vi "Initialize with Options.vi"(7 "Option string (\"\")":string, 8 "error in (no error)":errorcluster, 9 "Reset (T: Reset)":bool=TRUE, 10 "ID Query (T: Check)":bool=TRUE, 11 "VISA resource name":refnum<visa-resource-name>="TCPIP::192.168.5.120::INST") -> (0 "error out":errorcluster, 3 "VISA resource name out":refnum<visa-resource-name>)   [LabVIEW 2015, in "Rohde&Schwarz CMP LR WPAN Measurement.lvlib"]
doc: "This VI opens a new session to the instrument.\nCompared to the <b>Initialize.vi</b>, this one allows for additional settings in the <b>Option string</b>."
uses:
  <instrlib>/Rohde&Schwarz CMP LR WPAN Measurement/Rohde&Schwarz CMP LR WPAN Measurement.lvlib
  <instrlib>/Rohde&Schwarz CMP LR WPAN Measurement/Private/rsidr_core.llb/type_Session_Parameter_int32.ctl
  <instrlib>/Rohde&Schwarz CMP LR WPAN Measurement/Private/rsidr_core.llb/type_Session_Parameter_Boolean.ctl
  <instrlib>/Rohde&Schwarz CMP LR WPAN Measurement/Public/Utility/rsidr_core_global.vi
  <instrlib>/Rohde&Schwarz CMP LR WPAN Measurement/Private/rsidr_core.llb/rsidr_core.lvlib
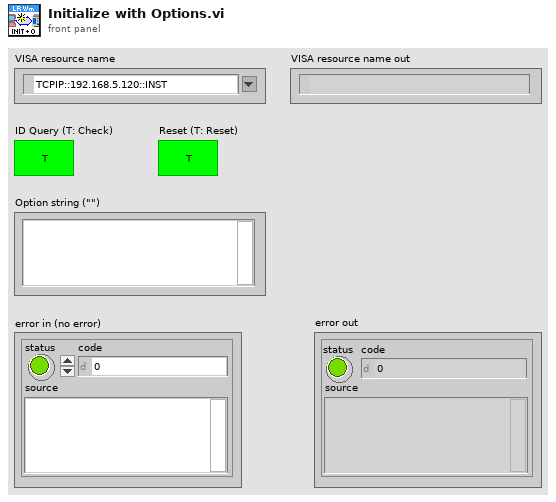
[diagram p1: front panel]
types:
  T1 = typedef "Rohde&Schwarz CMP LR WPAN Measurement.lvlib/rsidr_core.lvlib/type_Session_Parameter_Boolean.ctl" = enum16{"Simulate", "Query Instr Status", "Check Range", "Check Options", "Add LF to Write", "Duplicate Session", "Fast Sweep", "Logging", "OPC-sync Attribute Queries", "OPC-sync Attribute Writes"}
  T2 = typedef "Rohde&Schwarz CMP LR WPAN Measurement.lvlib/rsidr_core.lvlib/type_Session_Parameter_int32.ctl" = enum16{"OPC Timeout", "Additional Flags", "Wait Before Write", "Wait Before Read", "Bin Data Chunk Size", "VISA Access Mode", "VISA Timeout", "Bin Float Number Format", "Bin Integer Number Format", "STBpollVISAtimeout", "OPCwaitMode"}
  T3 = typedef "Rohde&Schwarz CMP LR WPAN Measurement.lvlib/rsidr_core.lvlib/type_Input_Format_RepCap.ctl" = cluster{"repCapName":string, "indetifiers":string[], "cmdValues":string[]}
  T4 = typedef "Rohde&Schwarz CMP LR WPAN Measurement.lvlib/rsidr_core.lvlib/type_Input_Format_RangeTable.ctl" = cluster{"Type":u16, "Name":string, "Entries":cluster{"Name":string, "Value 1":dbl, "Value 2":dbl, "Command":string}[]}
  T5 = typedef "Rohde&Schwarz CMP LR WPAN Measurement.lvlib/rsidr_core.lvlib/type_Input_Format_Attribute.ctl" = cluster{"Level":i32, "Class Only":bool, "Identifier":string, "Descriptive Name":string, "Data Type":u16, "Command":string, "Access":u16, "Range Table":string, "Read Callback":string, "Write Callback":string, "Supported Models":string, "Instrument Options":string, "Flags":i32, "Help":string}
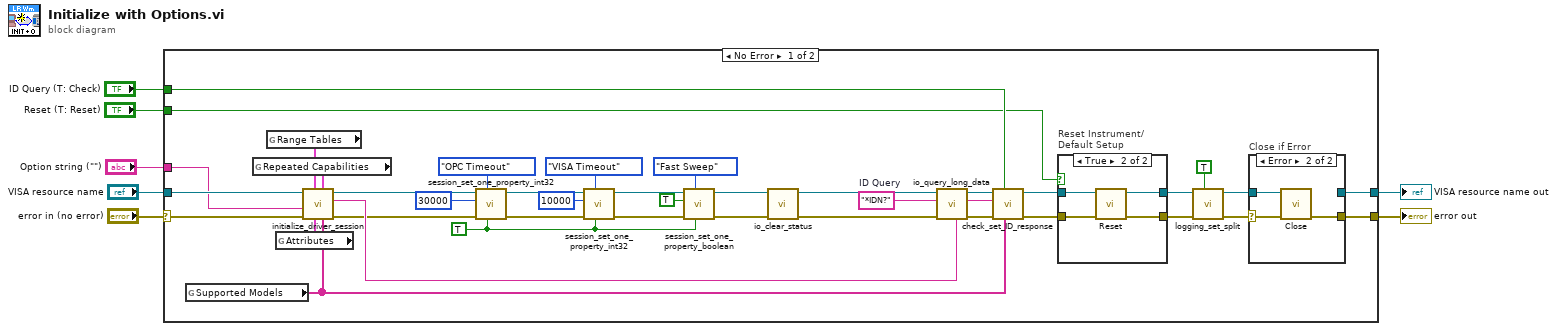
[diagram p0: block diagram]
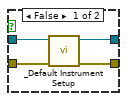
[diagram p3: hidden frame]
diagram:
  n1 = case shown="No Error" "error in (no error)" {
    selector: "error in (no error)" -> [w36 w61]
    tunnel: [w47 _] -> w7
    tunnel: [w37 w61] -> w6
    tunnel: "VISA resource name" -> [w35 _]
    tunnel: "Option string (\"\")" -> [w27 _]
    tunnel: "ID Query (T: Check)" -> [w26 _]
    tunnel: "Reset (T: Reset)" -> [w25 _]
    frame No Error {
      w10 = TRUE ("Skip setting if in option string (F)")
      w38 = "*IDN?"  # ID Query
      n2 = global read "rsidr_core_global.vi" "Supported Models"() -> (w29:string[])
      n3 = global read "rsidr_core_global.vi" "Repeated Capabilities"() -> (w43:T3[])
      n4 = global read "rsidr_core_global.vi" "Range Tables"() -> (w42:T4[])
      n5 = global read "rsidr_core_global.vi" "Attributes"() -> (w44:T5[])
      n6 = call <instrlib>:"initialize_driver_session.vi"("Supported instruments"=w29, "Repeated Capabilities"=w43, "Attributes"=w44, "Range Tables"=w42, "error in"=w36, "Option String"=w27, "VISA resource name"=w35) -> ("error out"=w21:errorcluster, "Simulation *IDN? response out"=w28:string, "VISA resource name out"=w20:refnum<visa-resource-name>)  [unwired: 2 in]
      n7 = call <instrlib>:"session_set_one_property_int32.vi"("Skip setting if in Options string (F)"=w10, "Session Parameter Integer"=type_Session_Parameter_int32."OPC Timeout" ("Session Parameter to set"), "error in"=w21, "Int32 value in"=30000 ("OPC Timeout"), "VISA resource name"=w20) -> ("error out"=w19:errorcluster, "VISA resource name out"=w18:refnum<visa-resource-name>)  [unwired: 4 in, 1 out]
      n8 = call <instrlib>:"session_set_one_property_int32.vi"("Skip setting if in Options string (F)"=w10, "Session Parameter Integer"=type_Session_Parameter_int32."VISA Timeout" ("Session Parameter to set"), "error in"=w19, "Int32 value in"=10000 ("int32 value in"), "VISA resource name"=w18) -> ("error out"=w16:errorcluster, "VISA resource name out"=w15:refnum<visa-resource-name>)  [unwired: 4 in, 1 out]
      n9 = call <instrlib>:"session_set_one_property_boolean.vi"("Skip setting if in Options string (F)"=w10, "Session Parameter Boolean"=type_Session_Parameter_Boolean."Fast Sweep" ("Session Parameter boolean"), "error in"=w16, "Boolean value in"=TRUE ("boolean value in"), "VISA resource name"=w15) -> ("error out"=w14:errorcluster, "VISA resource name out"=w13:refnum<visa-resource-name>)  [unwired: 4 in, 1 out]
      n10 = call <instrlib>:"io_clear_status.vi"("error in"=w14, "VISA resource name"=w13) -> ("error out"=w9:errorcluster, "VISA resource name out"=w8:refnum<visa-resource-name>)  [unwired: 8 in]
      n11 = call <instrlib>:"io_query_long_data.vi"("Simulation read buffer (\"Simulation\")"=w28, "error in"=w9, "write buffer"=w38, "VISA resource name"=w8) -> ("error out"=w41:errorcluster, "read buffer"=w39:string, "VISA resource name out"=w40:refnum<visa-resource-name>)  [unwired: 5 in]
      n12 = call <instrlib>:"check_set_ID_response.vi"("Supported instruments in"=w29, "Error if ID Query check fails"=w26, "error in"=w41, "IDN string in"=w39, "VISA resource name"=w40) -> ("error out"=w45:errorcluster, "VISA resource name out"=w46:refnum<visa-resource-name>)  [unwired: 3 in, 2 out]
      n13 = case "Reset Instrument/\nDefault Setup" shown="True" w25 {
        tunnel: w45 -> [w56 w60]
        tunnel: [w54 w59] -> w34
        tunnel: w46 -> [w55 w58]
        tunnel: [w53 w57] -> w33
        frame False {
          n14 = call <instrlib>:"_Default Instrument Setup.vi"("error in (no error)"=w56, "VISA resource name"=w55) -> ("error out"=w54:errorcluster, "VISA resource name out"=w53:refnum<visa-resource-name>)  [unwired: 8 in]
        }
        frame True {
          n15 = call <instrlib>:"Reset.vi"("error in (no error)"=w60, "VISA resource name"=w58) -> ("error out"=w59:errorcluster, "VISA resource name out"=w57:refnum<visa-resource-name>)  [unwired: 8 in]
        }
      }
      n16 = call <instrlib>:"logging_set_split.vi"("Evaluate section error (F)"=TRUE, "error in"=w34, "VISA resource name"=w33) -> ("error out"=w32:errorcluster, "VISA resource name out"=w31:refnum<visa-resource-name>)  [unwired: 7 in]
      n17 = case "Close if Error" shown="Error" w32 {
        selector: w32 -> [w48 w51]
        tunnel: w31 -> [w49 w52]
        tunnel: [w49 _] -> w47
        tunnel: [w48 w50] -> w37
        frame No Error {
        }
        frame Error {
          n18 = call <instrlib>:"Close.vi"("error in (no error)"=w51, "VISA resource name"=w52) -> ("error out"=w50:errorcluster)  [unwired: 9 in]
        }
      }
    }
    frame Error {
    }
  }
  "VISA resource name out" <- w7
  "error out" <- w6
